vi "Modbus Master.vi"(7 "error in":errorcluster, 8 "Unit ID":u8, 10 "holding register values":u16[](array[numeric]) caption="保持寄存器值", 11 "starting address":u16 caption="起始地址") -> (5 "error out":errorcluster)   [LabVIEW 2016]
uses:
  <vilib>/Modbus/subvis/Modbus API/Modbus API.lvclass/Modbus API.ctl
  <vilib>/Modbus/subvis/Transmission Data Unit (ADU)/Transmission Data Unit/Transmission Data Unit.lvclass/Transmission Data Unit.ctl
  <vilib>/Modbus/master/Data Access/Unit ID/Set Unit ID Property.vi
  <vilib>/Modbus/subvis/Transmission Data Unit (ADU)/Transmission Data Unit/Data Access/Unit ID/Write Unit ID.vi
  <vilib>/Modbus/subvis/Modbus API/Read Transmission Data Unit.vi
  <vilib>/Modbus/subvis/Modbus API/Write Transmission Data Unit.vi
  <vilib>/Modbus/master/Modbus Master.lvclass
  F:/Program Files/National Instruments/LabVIEW 2016/vi.lib/Modbus/subvis/Modbus API/Modbus API.lvclass
  <vilib>/Modbus/master/Create Master Instance (TCP).vi
  <vilib>/Modbus/subvis/Transmission Data Unit (ADU)/Transmission Data Unit/Transmission Data Unit.lvclass
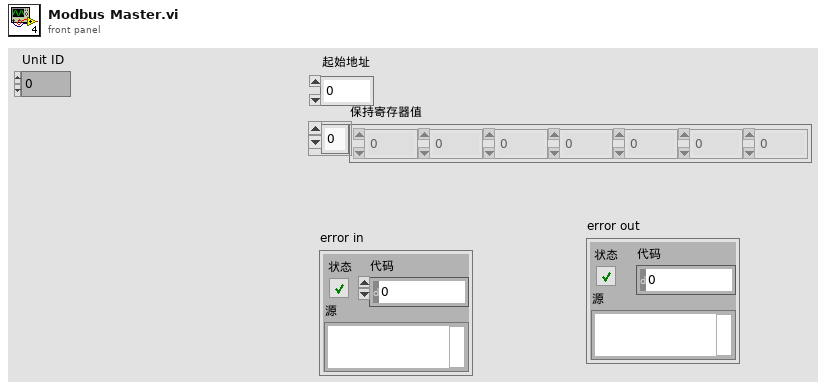
[diagram p1: front panel]
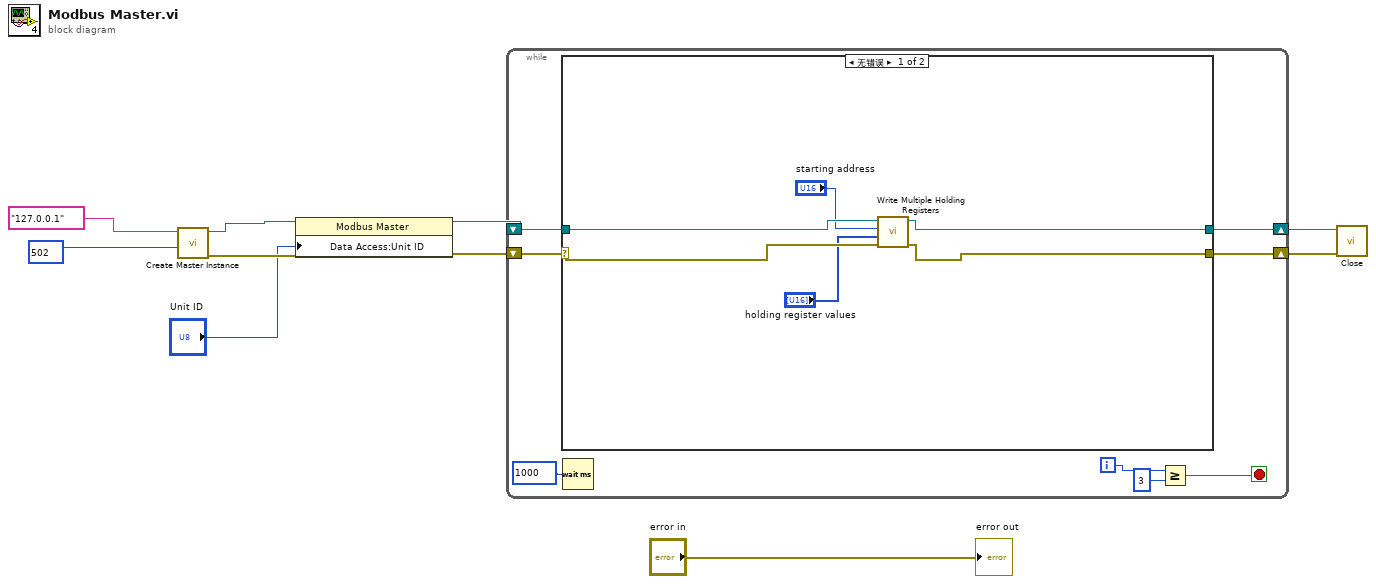
[diagram p0: block diagram]
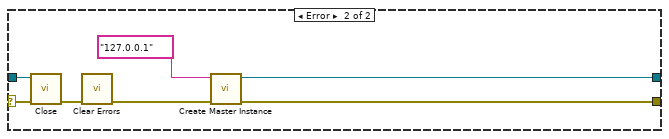
[diagram p2: hidden frame]
diagram:
  n1 = call-poly <vilib>:"Create Master Instance.vi"("port (502)"=u16 502, "address"="127.0.0.1") -> ("error out"=w9:errorcluster, "TCP master instance"=w4:refnum<class "Modbus Master.lvclass">)  [unwired: 8 in]
  n2 = property class="Modbus Master"(reference=w4, "Data Access:Unit ID"="Unit ID") -> (reference out=w3:refnum<class "Modbus Master.lvclass">)  [unwired: 1 in, 1 out]
  n3 = while {
    shift-right: [w15] -> w7
    shift-left: w9 -> [w14]
    shift-right: [w16] -> w8
    shift-left: w3 -> [w17]
    i -> [w12]
    stop <- w10 stop-if-true
    n4 = case shown="无错误" w14 {
      selector: w14 -> [w20 w29]
      tunnel: w17 -> [w23 w28]
      tunnel: [w22 w24] -> w16
      tunnel: [w21 w25] -> w15
      frame No Error {
        n5 = call-dynamic "Write Multiple Holding Registers.vi"("error in (no error)"=w20, "holding register values"="holding register values", "starting address"="starting address", "Modbus master in"=w23) -> ("error out"=w21:errorcluster, "Modbus master out"=w22:refnum<class "Modbus Master.lvclass">)  [unwired: 6 in]
      }
      frame Error {
        n6 = call-dynamic "Close.vi"("error in (no error)"=w29, "Modbus master in"=w28) -> ("error out"=w27:errorcluster)  [unwired: 9 in]
        n7 = call <vilib>:"Clear Errors.vi"("error in (no error)"=w27) -> ("error out"=w26:errorcluster)  [unwired: 5 in, 1 out]
        n8 = call-poly <vilib>:"Create Master Instance.vi"("error in (no error)"=w26, "address"="127.0.0.1") -> ("error out"=w25:errorcluster, "TCP master instance"=w24:refnum<class "Modbus Master.lvclass">)  [unwired: 8 in]
      }
    }
    n9 = Wait (ms)(milliseconds to wait=u32 1000 ("等待时间（毫秒）")) -> ()  [unwired: 1 out]
    n10 = Greater Or Equal?(x=w12, y=3) -> (x >= y?=w10:bool)
  }
  n11 = call-dynamic "Close.vi"("error in (no error)"=w7, "Modbus master in"=w8) -> ()  [unwired: 9 in, 1 out]
  "error out" <- "error in"
